vi "Forward Packet.vi"(10 "Response":T1, 11 "Session in":refnum<class "Session.lvclass">) -> (0 "error out":errorcluster)   [LabVIEW 2013, in "MQTT Base.lvlib" / "Session.lvclass"]
uses:
  Session.lvclass
  Base Class/Response -- cluster.ctl
  <vilib>/LabVIEW Open Source Project/MQTT Control Packets/Control Packets/ControlPacket/ControlPacket.lvclass
  Pending ACKs -- cluster.ctl
  <vilib>/LabVIEW Open Source Project/MQTT Control Packets/Control Packets/ControlPacket/ControlPacket.lvclass/ControlPacket.ctl
  Session.lvclass/Session.ctl
  MQTT_Connection/Connection/Connection.lvclass
  Base Class/MQTT_Base.lvclass
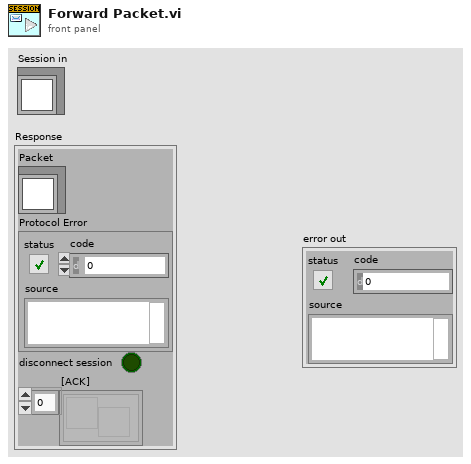
[diagram p1: front panel]
types:
  T1 = typedef "MQTT Base.lvlib/MQTT_Base.lvclass/Response -- cluster.ctl" = cluster{"Packet":refnum<class "ControlPacket.lvclass">, "Protocol Error":errorcluster, "disconnect session":bool, "[ACK]":refnum<notifier>[]}
  T2 = typedef "MQTT Base.lvlib/Session.lvclass/Pending ACKs -- cluster.ctl" = cluster{"Message":refnum<class "ControlPacket.lvclass">, "[ACK]":refnum<notifier>[], "Packet Identifier":u16}
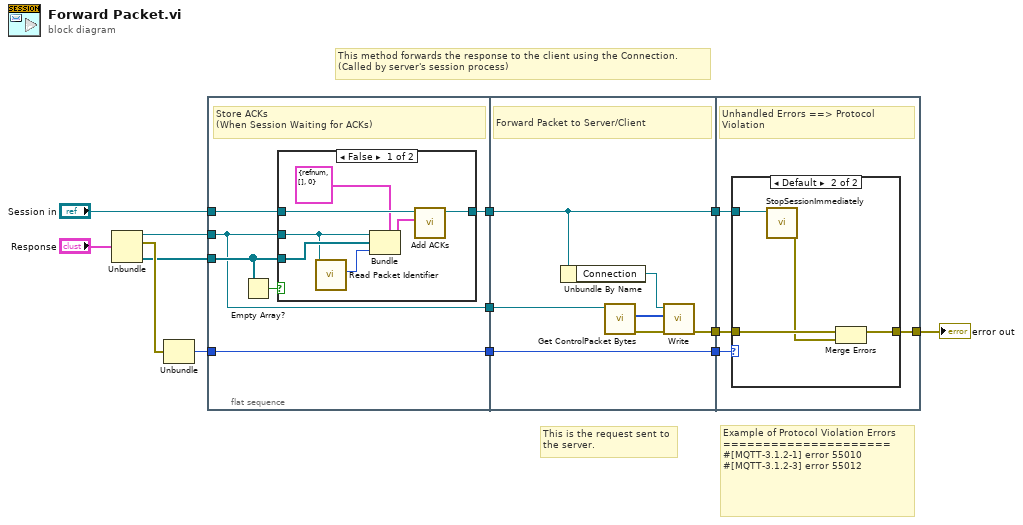
[diagram p0: block diagram]
diagram:
  # "This is the request sent to\nthe server."
  # "Example of Protocol Violation Errors\n=====================\n#[MQTT-3.1.2-1] error 55010\n#[MQTT-3.1.2-3] error 55012"
  # "This method forwards the response to the client using the Connection.\n(Called by server's session process)"
  n1 = Unbundle("Response") -> ("Packet"=w7:refnum<class "ControlPacket.lvclass">, "Protocol Error"=w6:errorcluster, "[ACK]"=w5:refnum<notifier>[])  [unwired: 1 out]
  n2 = Unbundle(w6) -> ("code"=w1:i32)  [unwired: 2 out]
  n3 = flat-sequence {
    tunnel: w1 -> [w19]
    tunnel: "Session in" -> [w18]
    tunnel: w7 -> [w14]
    tunnel: [w19] -> w13
    tunnel: w5 -> [w15]
    tunnel: [w16] -> w12
    tunnel: [w14] -> w11
    tunnel: [w29] -> w10
    tunnel: [w33] -> w9
    tunnel: [w32] -> w8
    tunnel: w13 -> [w33]
    tunnel: w12 -> [w32]
    tunnel: w11 -> [w34]
    tunnel: [w35] -> w2
    tunnel: w10 -> [w36]
    tunnel: w9 -> [w37]
    tunnel: w8 -> [w38]
    frame #0 {
      # "Store ACKs\n(When Session Waiting for ACKs)"
      n4 = Empty Array?(array=w15) -> (empty?=w17:bool)
      n5 = case shown="False" w17 {
        tunnel: w18 -> [w26 w27]
        tunnel: [w25 w27] -> w16
        tunnel: w14 -> [w22 _]
        tunnel: w15 -> [w24 _]
        frame False {
          n6 = call <vilib>:"Read Packet Identifier.vi"("ControlPacket in"=w22) -> ("Packet Identifier"=w21:u16)  [unwired: 9 in, 1 out]
          n7 = Bundle(cluster=T2 {"Message"=refnum, "[ACK]"=[], "Packet Identifier"=0} ("Pending ACK"), "Message"=w22, "[ACK]"=w24, "Packet Identifier"=w21) -> (w23:T2)
          n8 = call "Add ACKs.vi"("Pending ACK"=w23, "Session in"=w26) -> ("Session out"=w25:refnum<class "Session.lvclass">)  [unwired: 8 in, 1 out]
        }
        frame True {
          # "No Acks."
        }
      }
    }
    frame #1 {
      # "Forward Packet to Server/Client"
      n9 = Unbundle By Name(w32) -> ("Connection"=w31:refnum<class "Connection.lvclass">)
      n10 = call <vilib>:"Get ControlPacket Bytes.vi"("ControlPacket"=w34) -> ("error out"=w30:errorcluster, "Bytes Stream"=w28:u8[])  [unwired: 7 in, 2 out]
      n11 = call "Write.vi"("error in (no error)"=w30, "Bytes"=w28, "Connection in"=w31) -> ("error out"=w29:errorcluster)  [unwired: 7 in, 1 out]
    }
    frame #2 {
      # "Unhandled Errors ==> Protocol Violation"
      n12 = case shown="Default" w37 {
        tunnel: w38 -> [_ w43]
        tunnel: w36 -> [w39 w42]
        tunnel: [w39 w40] -> w35
        frame 0 {
        }
        frame Default {
          n13 = call "StopSessionImmediately.vi"("Session in"=w43) -> ("error out"=w41:errorcluster)  [unwired: 9 in, 1 out]
          n14 = Merge Errors(w42, w41) -> (w40:errorcluster)
        }
      }
    }
  }
  "error out" <- w2
